vi "RunTimeMenu_Add_Current_Chan.vi"(8 "error in (no error)":errorcluster, 11 "Node Ptr":u64 format="%.0x") -> (0 "error out":errorcluster)   [LabVIEW 2018, in "NI PXI-4110 Programmable Power Supply Custom Device.lvlib"]
uses:
  NI PXI-4110 Programmable Power Supply Custom Device.lvlib
  4110_Global.vi
  <vilib>/NI Veristand/Custom Device API/Get Item Property (U16).vi
  <vilib>/NI VeriStand/Custom Device API/Custom Device API.lvlib
panel:
  in  "Tag":string
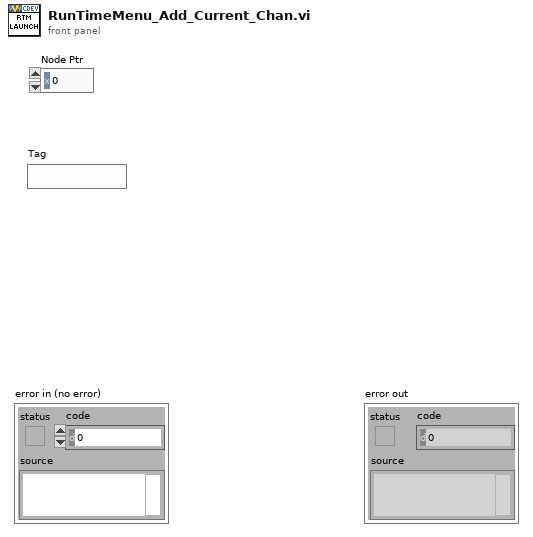
[diagram p1: front panel]
types:
  T1 = typedef "Custom Device API.lvlib/Custom Device Item Ref.ctl" = u64
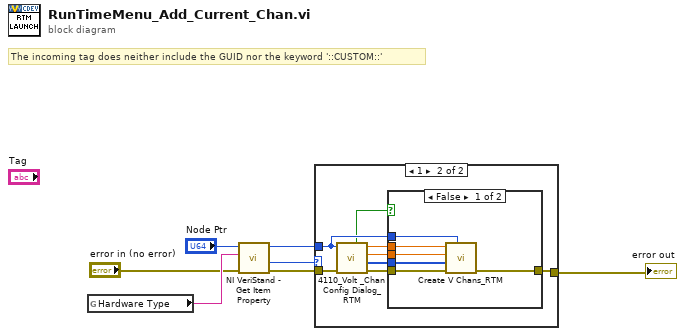
[diagram p0: block diagram]
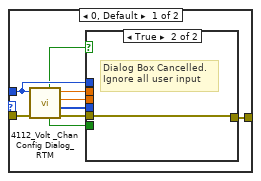
[diagram p2: hidden frame]
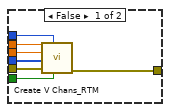
[diagram p3: hidden frame]
diagram:
  # "The incoming tag does neither include the GUID nor the keyword '::CUSTOM::'"
  n1 = global read "4110_Global.vi" "Hardware Type"() -> (w4:string)
  n2 = call-poly <vilib>:"NI VeriStand - Get Item Property.vi"("error in (no error)"="error in (no error)", "Property Name"=w4, "Item Ref in"="Node Ptr") -> ("error out"=w7:errorcluster, "Value"=w5:u16, "Item Ref out"=w6:T1)  [unwired: 5 in, 1 out]
  n3 = case shown="1" w5 {
    tunnel: w6 -> [w15 w27]
    tunnel: w7 -> [w16 w32]
    tunnel: [w8 w25] -> w1
    frame 0, Default {
      n4 = call "4112_Volt _Chan Config Dialog_RTM.vi"("error in (no error)"=w16, "CD PTR"=w15) -> ("error out"=w12:errorcluster, "Channels to Add"=w10:u16[], "Current Limit (out)"=w11:dbl, "Initial Voltage Value (out)"=w13:dbl, "Remote Sense?"=w9:bool, "Cancel (out)"=w14:bool)  [unwired: 4 in]
      n5 = case shown="True" w14 {
        tunnel: w15 -> [w23 _]
        tunnel: w13 -> [w22 _]
        tunnel: w12 -> [w21 w24]
        tunnel: w11 -> [w20 _]
        tunnel: w10 -> [w19 _]
        tunnel: w9 -> [w18 _]
        tunnel: [w17 w24] -> w8
        frame False {
          n6 = call "Create V Chans_RTM.vi"("Remote Sense?"=w18, "Device Ref in"=w23, "error in"=w21, "Channels to Add"=w19, "Current Limit"=w20, "Init Value"=w22) -> ("error out"=w17:errorcluster)  [unwired: 5 in]
        }
        frame True {
          # "Dialog Box Cancelled.\nIgnore all user input"
        }
      }
    }
    frame 1 {
      n7 = call "4110_Volt _Chan Config Dialog_RTM.vi"("error in (no error)"=w32, "CD PTR"=w27) -> ("error out"=w30:errorcluster, "Channels to Add"=w31:u16[], "Current Limit (out)"=w28:dbl, "Initial Voltage Value (out)"=w29:dbl, "Cancel (out)"=w26:bool)  [unwired: 5 in]
      n8 = case shown="False" w26 {
        tunnel: w31 -> [w37 _]
        tunnel: w30 -> [w38 w39]
        tunnel: w29 -> [w36 _]
        tunnel: w28 -> [w35 _]
        tunnel: w27 -> [w34 _]
        tunnel: [w33 w39] -> w25
        frame False {
          n9 = call "Create V Chans_RTM.vi"("Device Ref in"=w34, "error in"=w38, "Channels to Add"=w37, "Current Limit"=w35, "Init Value"=w36) -> ("error out"=w33:errorcluster)  [unwired: 6 in]
        }
        frame True {
          # "Dialog Box Cancelled.\nIgnore all user input"
        }
      }
    }
  }
  "error out" <- w1
